vi "tabla de multiplicar.vi"() -> ()   [LabVIEW 2020]
panel:
  in  "Filas":i32
  in  "Columnas":i32
  out "element":i32
  in  "Columna":i32
  in  "Fila":i32
  out "Array":dbl[][](array[numeric])
  # "Generar Tabla"
  # "Obtener multiplicacion"
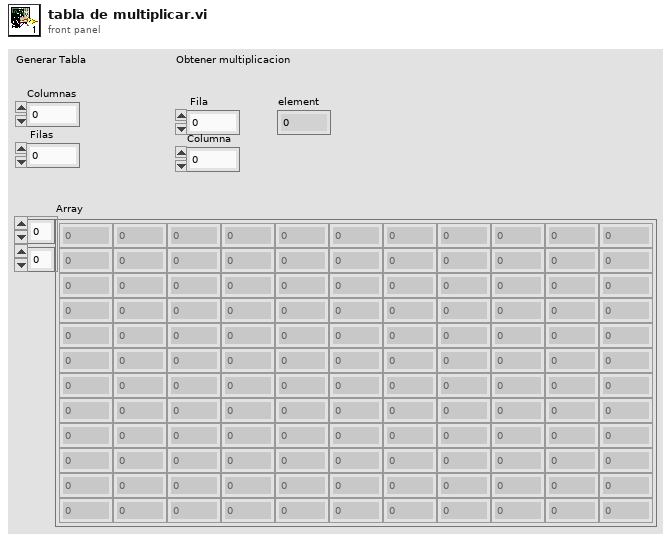
[diagram p1: front panel]
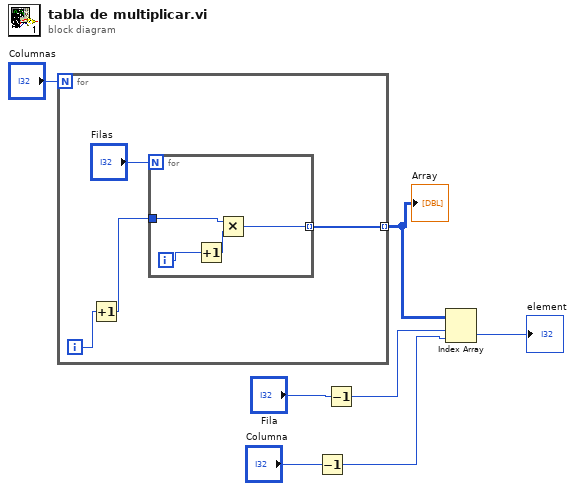
[diagram p0: block diagram]
diagram:
  n1 = for {
    N: "Columnas" -> [_]
    tunnel: [w11] -> w7 mode=indexing
    i -> [w10]
    n2 = Increment(x=w10) -> (x+1=w9:i32)
    n3 = for {
      N: "Filas" -> [_]
      tunnel: [w15] -> w11 mode=indexing
      tunnel: w9 -> [w12]
      i -> [w14]
      n4 = Increment(x=w14) -> (x+1=w13:i32)
      n5 = Multiply(x=w12, y=w13) -> (x*y=w15:i32)
    }
  }
  "Array" <- w7
  n6 = Decrement(x="Columna") -> (x-1=w2:i32)
  n7 = Decrement(x="Fila") -> (x-1=w4:i32)
  n8 = Index Array(array=w7, index (row)=w4, index (col)=w2) -> (element=→"element":i32)
